vi "Handle UNSUBSCRIBED.vi"(8 "error in (no error)":errorcluster, 9 "Message Loop data (in)":T1, 10 "WAMP Message":T16 {"Message Codes" items=["HELLO"=1, "WELCOME"=2, "ABORT"=3, "GOODBYE"=6, "ERROR"=8, "PUBLISH"=16, "PUBLISHED"=17, "SUBSCRIBE"=32, "SUBSCRIBED"=33, "UNSUBSCRIBE"=34, "UNSUBSCRIBED"=35, "EVENT"=36, "CALL"=48, "RESULT"=59, "REGISTER"=64, "REGISTERED"=65, "UNREGISTER"=66, "UNREGISTERED"=67, "INVOCATION"=68, "YIELD"=70]}, 11 "reference":refnum<class "WAMP Client.lvclass">) -> (0 "error out":errorcluster, 1 "Message Loop Data (Out)":T1, 3 "reference out":refnum<class "WAMP Client.lvclass">)   [LabVIEW 2020, in "wamplv.lvlib" / "WAMP Client.lvclass"]
uses:
  WAMP Client.lvclass
  TypeDef/WAMP Received Message.ctl
  TypeDef/WAMP Message Codes.ctl
  TypeDef/Message Loop Shift Reg Data.ctl
  TypeDef/REGISTER Request Data.ctl
  API/TypeDefs/INVOCATION payload.ctl
  TypeDef/Success or error.ctl
  API/TypeDefs/Combined error.ctl
  API/TypeDefs/WAMP error.ctl
  TypeDef/Publish Requests Map.ctl
  TypeDef/PUBLISH Request Data.ctl
  TypeDef/PUBLISH result.ctl
  TypeDef/Endpoint Data.ctl
  TypeDef/CALL Request Map.ctl
  TypeDef/CALL Request Data.ctl
  API/TypeDefs/RESULT payload.ctl
  TypeDef/SUBSCRIBE Requests Map.ctl
  TypeDef/SUBSCRIBE Request Data.ctl
  TypeDef/Subscribe Result.ctl
  TypeDef/EVENT payload.ctl
  TypeDef/Subscriptions Map.ctl
  TypeDef/Subscription Details.ctl
  TypeDef/Unsubscribe Requests Map.ctl
  TypeDef/UNSUBSCRIBE Request Data.ctl
  TypeDef/UNSUBSCRIBE Result.ctl
  TypeDef/Unregister requests map.ctl
  TypeDef/Unregister request.ctl
  73a204a7-fc9f-47f9-93b3-f48d89583bd3.vi
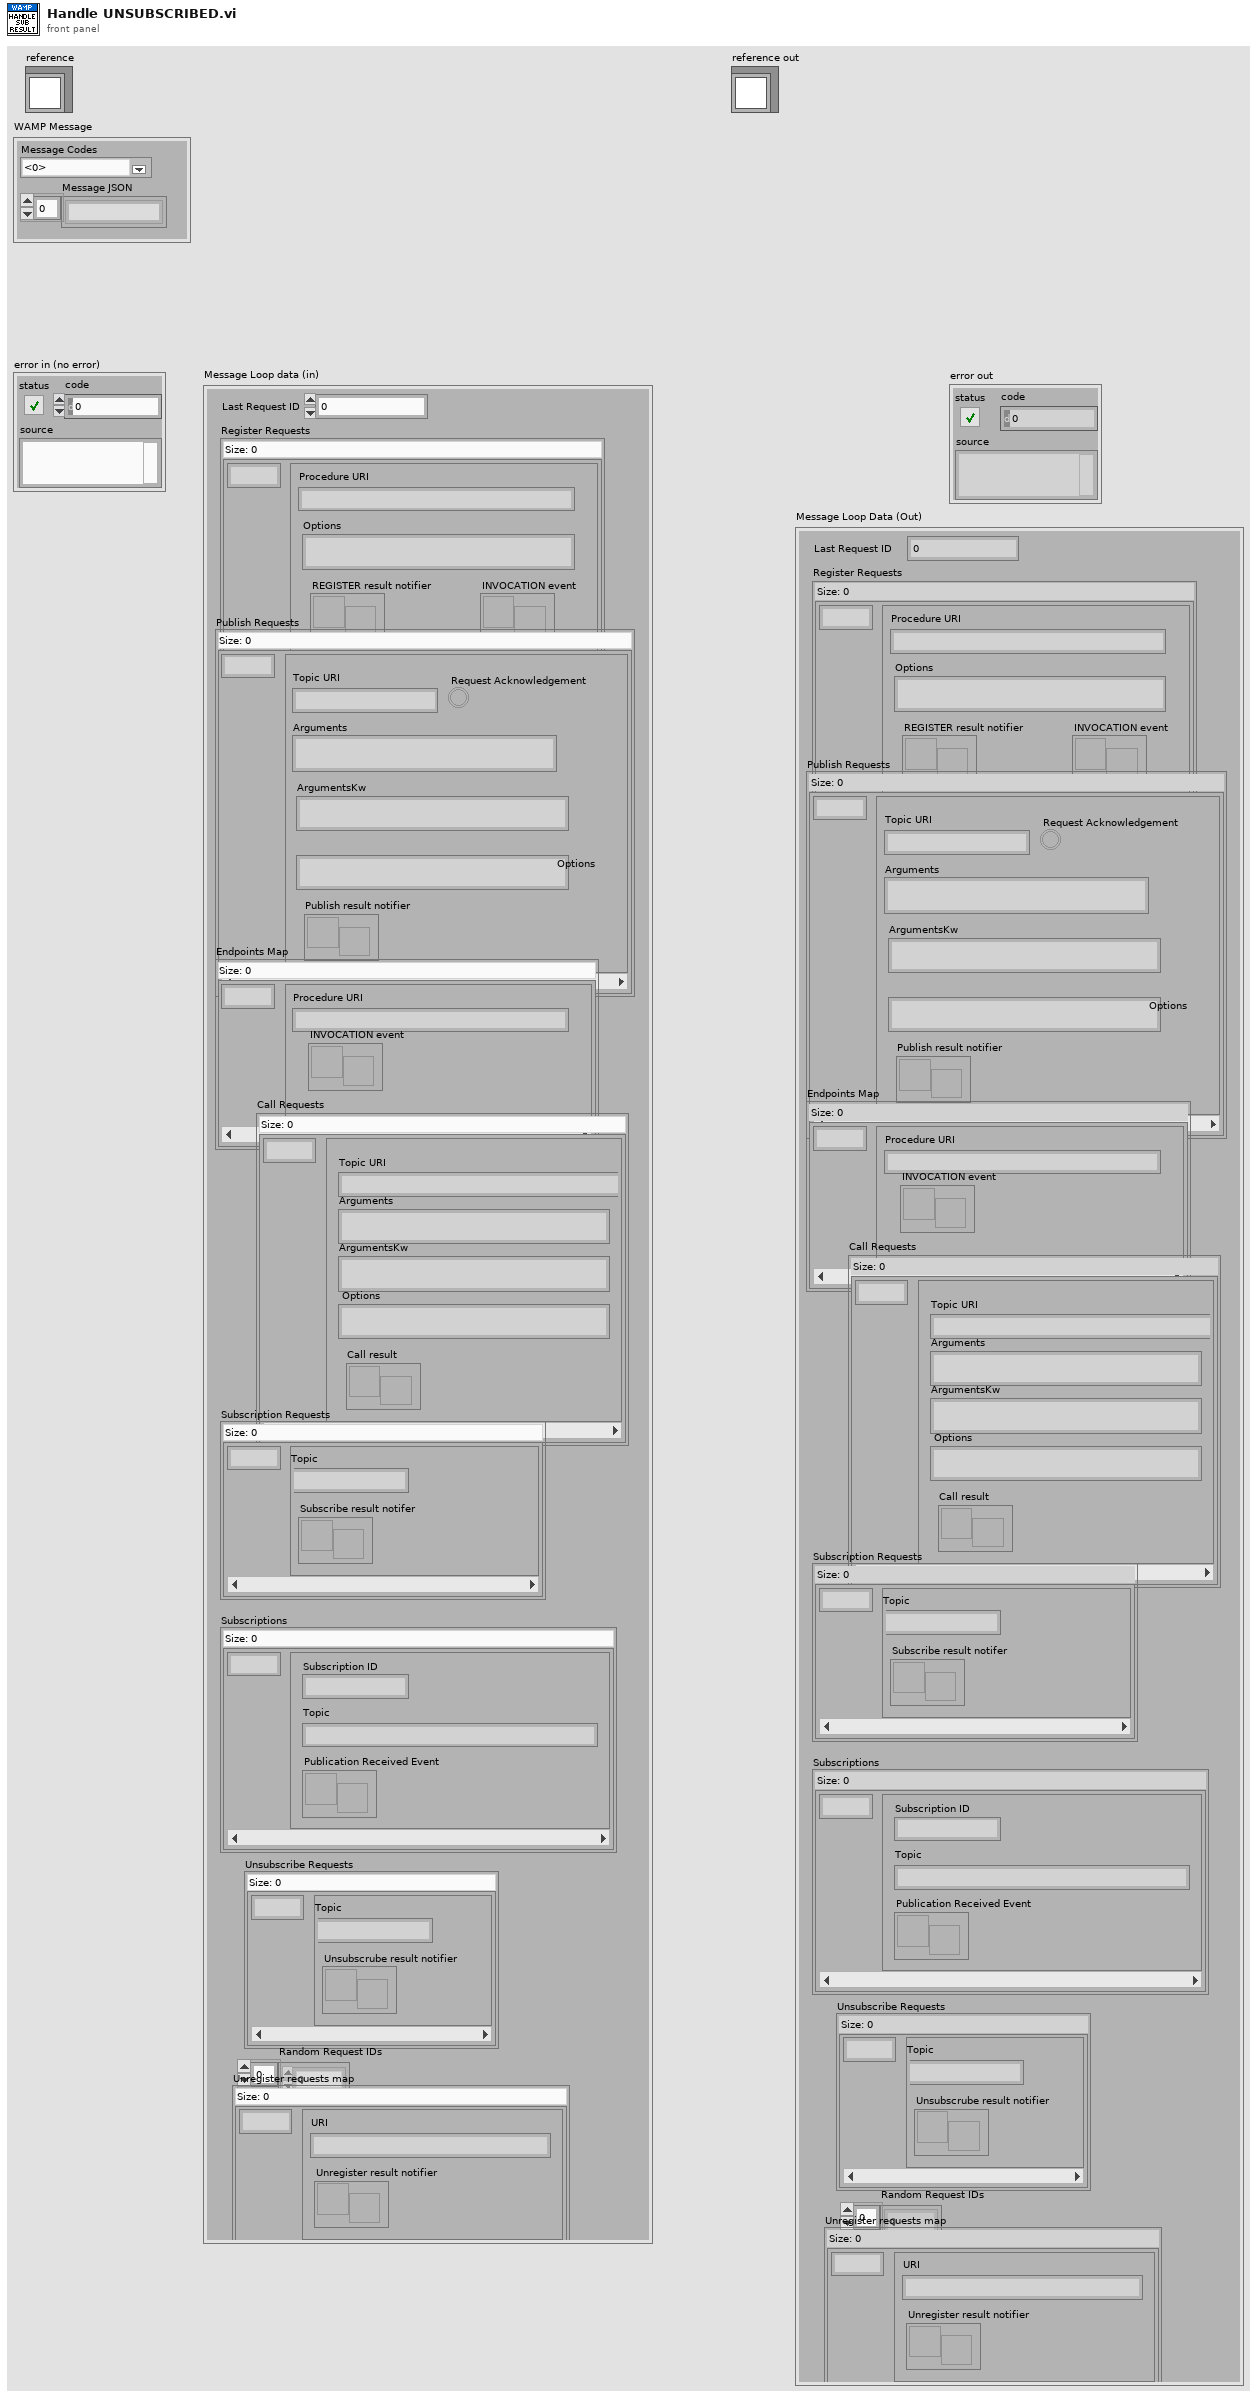
[diagram p1: front panel]
types:
  T1 = typedef "wamplv.lvlib/WAMP Client.lvclass/Message Loop Shift Reg Data.ctl" = cluster{"Last Request ID":u64, "Register Requests":map{u64, T2}, "Publish Requests":T3, "Endpoints Map":map{u64, T5}, "Call Requests":T6, "Subscription Requests":T8, "Subscriptions":T10, "Unsubscribe Requests":T12, "Random Request IDs":u64[], "Unregister requests map":T14}
  T2 = typedef "wamplv.lvlib/WAMP Client.lvclass/REGISTER Request Data.ctl" = cluster{"Procedure URI":string, "Options":string, "INVOCATION event":refnum<user-event>, "REGISTER result notifier":refnum<notifier>}
  T3 = typedef "wamplv.lvlib/WAMP Client.lvclass/Publish Requests Map.ctl" = map{u64, T4}
  T4 = typedef "wamplv.lvlib/WAMP Client.lvclass/PUBLISH Request Data.ctl" = cluster{"Topic URI":string, "Arguments":string, "ArgumentsKw":string, "Request Acknowledgement":bool, "Options":string, "Publish result notifier":refnum<notifier>}
  T5 = typedef "wamplv.lvlib/WAMP Client.lvclass/Endpoint Data.ctl" = cluster{"Procedure URI":string, "INVOCATION event":refnum<user-event>}
  T6 = typedef "wamplv.lvlib/WAMP Client.lvclass/CALL Request Map.ctl" = map{u64, T7}
  T7 = typedef "wamplv.lvlib/WAMP Client.lvclass/CALL Request Data.ctl" = cluster{"Topic URI":string, "Arguments":string, "ArgumentsKw":string, "Options":string, "Call result":refnum<notifier>}
  T8 = typedef "wamplv.lvlib/WAMP Client.lvclass/SUBSCRIBE Requests Map.ctl" = map{u64, T9}
  T9 = typedef "wamplv.lvlib/WAMP Client.lvclass/SUBSCRIBE Request Data.ctl" = cluster{"Topic":string, "Subscribe result notifer":refnum<notifier>}
  T10 = typedef "wamplv.lvlib/WAMP Client.lvclass/Subscriptions Map.ctl" = map{u64, T11}
  T11 = typedef "wamplv.lvlib/WAMP Client.lvclass/Subscription Details.ctl" = cluster{"Subscription ID":u64, "Topic":string, "Publication Received Event":refnum<user-event>}
  T12 = typedef "wamplv.lvlib/WAMP Client.lvclass/Unsubscribe Requests Map.ctl" = map{u64, T13}
  T13 = typedef "wamplv.lvlib/WAMP Client.lvclass/UNSUBSCRIBE Request Data.ctl" = cluster{"Topic":string, "Unsubscrube result notifier":refnum<notifier>}
  T14 = typedef "wamplv.lvlib/WAMP Client.lvclass/Unregister requests map.ctl" = map{u64, T15}
  T15 = typedef "wamplv.lvlib/WAMP Client.lvclass/Unregister request.ctl" = cluster{"URI":string, "Unregister result notifier":refnum<notifier>}
  T16 = typedef "wamplv.lvlib/WAMP Client.lvclass/WAMP Received Message.ctl" = cluster{"Message JSON":string[], "Message Codes":T17}
  T17 = typedef "wamplv.lvlib/WAMP Client.lvclass/WAMP Message Codes.ctl" = u16
  T18 = typedef "wamplv.lvlib/WAMP Client.lvclass/UNSUBSCRIBE Result.ctl" = cluster{"Success?":bool, "Combined Error":T19}
  T19 = typedef "wamplv.lvlib/WAMP Client.lvclass/Combined error.ctl" = cluster{"Error?":bool, "WAMP Error":T20, "Error":errorcluster}
  T20 = typedef "wamplv.lvlib/WAMP Client.lvclass/WAMP error.ctl" = cluster{"Details":string, "ArgumentKw Payload":string, "Error?":bool, "Error URI":string, "Arguments Payload":string}
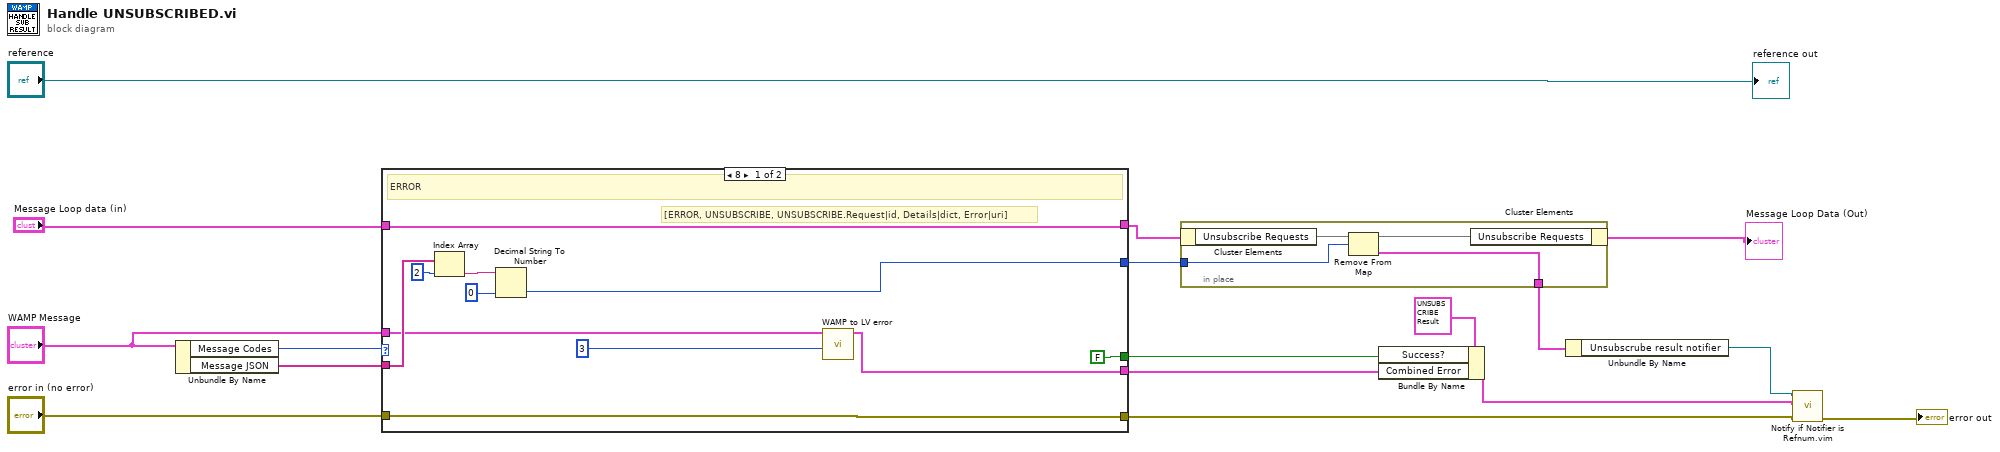
[diagram p0: block diagram]
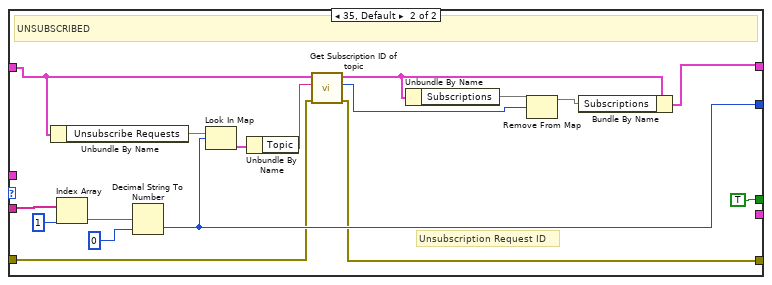
[diagram p2: hidden frame]
diagram:
  n1 = Unbundle By Name("WAMP Message") -> ("Message Codes"=w13:T17, "Message JSON"=w12:string[])
  n2 = case shown="8" w13 {
    tunnel: w12 -> [w26 w38]
    tunnel: [w24 w36] -> w11
    tunnel: "error in (no error)" -> [w25 w30]
    tunnel: [w25 w29] -> w6
    tunnel: [w18 _] -> w16
    tunnel: [FALSE ("Success?") TRUE ("Success?")] -> w15
    tunnel: "Message Loop data (in)" -> [w23 w33]
    tunnel: [w23 w39] -> w2
    tunnel: "WAMP Message" -> [w20 _]
    frame 8 {
      # "[ERROR, UNSUBSCRIBE, UNSUBSCRIBE.Request|id, Details|dict, Error|uri]"
      # "ERROR"
      n3 = Index Array(array=w26, index=2) -> (element=w27:string)
      n4 = Decimal String To Number(string=w27, default (0L)=u64 0 ("default (0 I32)")) -> (number=w24:u64)  [unwired: 1 in, 1 out]
      n5 = call "WAMP to LV error.vi"("Details Index"=u32 3, "WAMP Message"=w20) -> ("Combined Error"=w18:T19)  [unwired: 7 in, 2 out]
    }
    frame 35, Default {
      # "Unsubscription Request ID"
      # "UNSUBSCRIBED"
      n6 = Unbundle By Name(w33) -> ("Unsubscribe Requests"=w37:T12)
      n7 = Index Array(array=w38, index=1) -> (element=w43:string)
      n8 = Decimal String To Number(string=w43, default (0L)=u64 0) -> (number=w36:u64)  [unwired: 1 in, 1 out]
      n9 = Look In Map(map=w37, key=w36) -> (value=w35:T13)  [unwired: 1 in, 1 out]
      n10 = Unbundle By Name(w35) -> ("Topic"=w34:string)
      n11 = call "Get Subscription ID of topic.vi"("error in"=w30, "Topic"=w34, "Message loop data (in)"=w33) -> ("error out"=w29:errorcluster, "Subscriiiption ID"=w31:u64, "Message loop data (out)"=w32:T1)  [unwired: 6 in]
      n12 = Unbundle By Name(w32) -> ("Subscriptions"=w41:T10)
      n13 = Remove From Map(10:w31, 11:w41) -> (3:w40:T10)  [unwired: 2 out]
      n14 = Bundle By Name(cluster=w32, "Subscriptions"=w40) -> (w39:T1)
    }
  }
  n15 = in-place {
    in-place-border: w11 -> [w49]
    in-place-border: [w48] -> w10
    n16 = in-place-cluster #1(w2) -> ("Unsubscribe Requests"=w47:T12)
    n17 = Remove From Map(10:w49, 11:w47) -> (1:w48:T13, 3:w46:T12)  [unwired: 1 out]
    n18 = in-place-cluster #1("Unsubscribe Requests"=w46) -> (→"Message Loop Data (Out)":T1)
  }
  n19 = Bundle By Name(cluster=T18 {"Success?"=FALSE, "Combined Error"={"Error?"=FALSE, "WAMP Error"={"Details"="", "ArgumentKw Payload"="{}", "Error?"=FALSE, "Error URI"="", "Arguments Payload"=""}, "Error"={"status"=FALSE, "code"=0, "source"=""}}} ("Unsubcsribe Result"), "Success?"=w15, "Combined Error"=w16) -> (w5:T18)
  n20 = Unbundle By Name(w10) -> ("Unsubscrube result notifier"=w4:refnum<notifier>)
  n21 = call "Notify if Notifier is Refnum.vim"("error in (no error)"=w6, "RESULT Payload"=w5, "Notifier in"=w4) -> ("error out"=→"error out":errorcluster)  [unwired: 8 in]
  "reference out" <- "reference"
